vi "Limit.vi"(10 "string array":string[](array[string]), 11 "Enum":T1(ring)) -> (2 "Limits 2":dbl[](array[numeric]), 3 "Limits":dbl[](array[numeric]))   [LabVIEW 2021]
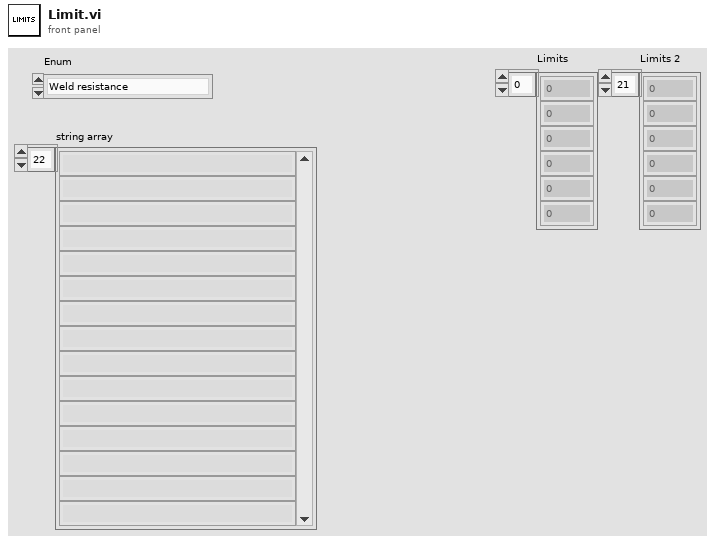
[diagram p1: front panel]
types:
  T1 = enum16{"Weld resistance", "Voltage", "Voltage befor WR", "Temp"}
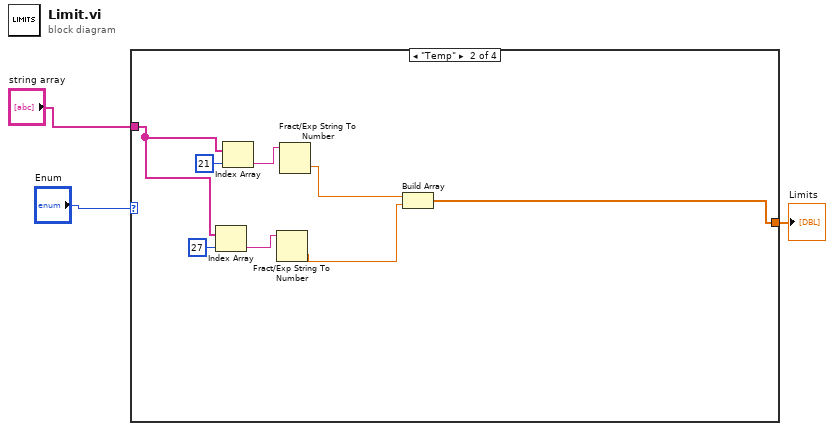
[diagram p0: block diagram]
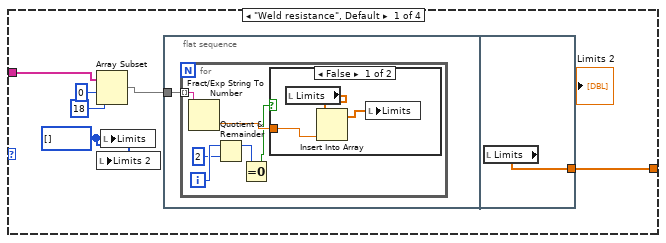
[diagram p2: hidden frame]
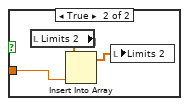
[diagram p3: hidden frame]
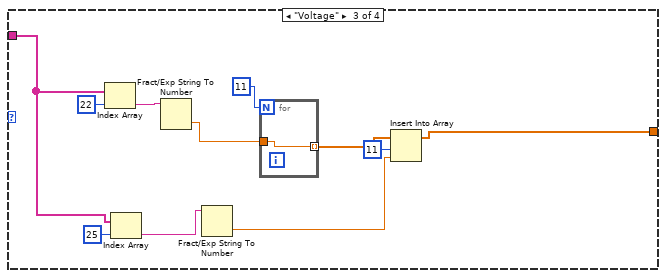
[diagram p4: hidden frame]
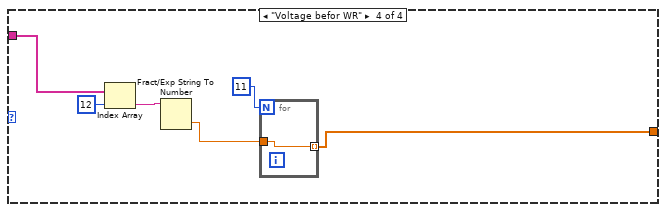
[diagram p5: hidden frame]
diagram:
  n1 = case shown="\"Temp\"" "Enum" {
    tunnel: "string array" -> [w6 w27 w42 w49]
    tunnel: [w5 w24 w32 w44] -> w1
    frame "Weld resistance", Default {
      w4 = i32[] [] ("Limits")
      n2 = Array Subset(array=w6, index=0, length=18) -> (w7:string[])
      n3 = local write "Limits 2"(w4) -> ()
      n4 = local write "Limits"(w4) -> ()
      n5 = flat-sequence {
        tunnel: w7 -> [w10]
        tunnel: [w23] -> w5
        frame #0 {
          n6 = for {
            tunnel: w10 -> [w16] mode=indexing
            i -> [w14]
            n7 = Fract/Exp String To Number(string=w16) -> (number=w15:dbl)  [unwired: 3 in, 1 out]
            n8 = Quotient & Remainder(x=w14, y=2) -> (x-y*floor(x/y)=w12:i32)  [unwired: 1 out]
            n9 = Equal To 0?(x=w12) -> (x = 0?=w11:bool)
            n10 = case shown="False" w11 {
              tunnel: w15 -> [w17 w20]
              frame False {
                n11 = local read "Limits"() -> (w19:dbl[])
                n12 = Insert Into Array(array=w19, new element=w17) -> (w18:dbl[])  [unwired: 1 in]
                n13 = local write "Limits"(w18) -> ()
              }
              frame True {
                n14 = local read "Limits 2"() -> (w22:dbl[])
                n15 = Insert Into Array(array=w22, new element=w20) -> (w21:dbl[])  [unwired: 1 in]
                n16 = local write "Limits 2"(w21) -> ()
              }
            }
          }
        }
        frame #1 {
          n17 = local read "Limits"() -> (w23:dbl[])
        }
      }
    }
    frame "Temp" {
      n18 = Index Array(array=w27, index=27) -> (element=w28:string)
      n19 = Index Array(array=w27, index=21) -> (element=w29:string)
      n20 = Fract/Exp String To Number(string=w28) -> (number=w26:dbl)  [unwired: 3 in, 1 out]
      n21 = Fract/Exp String To Number(string=w29) -> (number=w25:dbl)  [unwired: 3 in, 1 out]
      n22 = Build Array(w25, w26) -> (w24:dbl[])
    }
    frame "Voltage" {
      n23 = Index Array(array=w42, index=22) -> (element=w38:string)
      n24 = Index Array(array=w42, index=25) -> (element=w39:string)
      n25 = Fract/Exp String To Number(string=w38) -> (number=w37:dbl)  [unwired: 3 in, 1 out]
      n26 = Fract/Exp String To Number(string=w39) -> (number=w34:dbl)  [unwired: 3 in, 1 out]
      n27 = for {
        N: 11 -> [_]
        tunnel: w37 -> [w43]
        tunnel: [w43] -> w35 mode=indexing
      }
      n28 = Insert Into Array(array=w35, index=11, new element=w34) -> (w32:dbl[])
    }
    frame "Voltage befor WR" {
      n29 = Index Array(array=w49, index=12) -> (element=w47:string)
      n30 = Fract/Exp String To Number(string=w47) -> (number=w46:dbl)  [unwired: 3 in, 1 out]
      n31 = for {
        N: 11 -> [_]
        tunnel: w46 -> [w50]
        tunnel: [w50] -> w44 mode=indexing
      }
    }
  }
  "Limits" <- w1
